vi "9149_9205_AI_64.vi"() -> (3 "Array":fxp<+/-,26,5>[](array[numeric]))   [LabVIEW 2017]
uses:
  <vilib>/rvi/eio/common/nirviEmuTemplateMethod_errors.vi
  <vilib>/eio/EIONode/EIONode.xnode
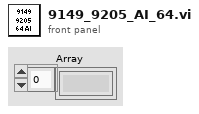
[diagram p1: front panel]
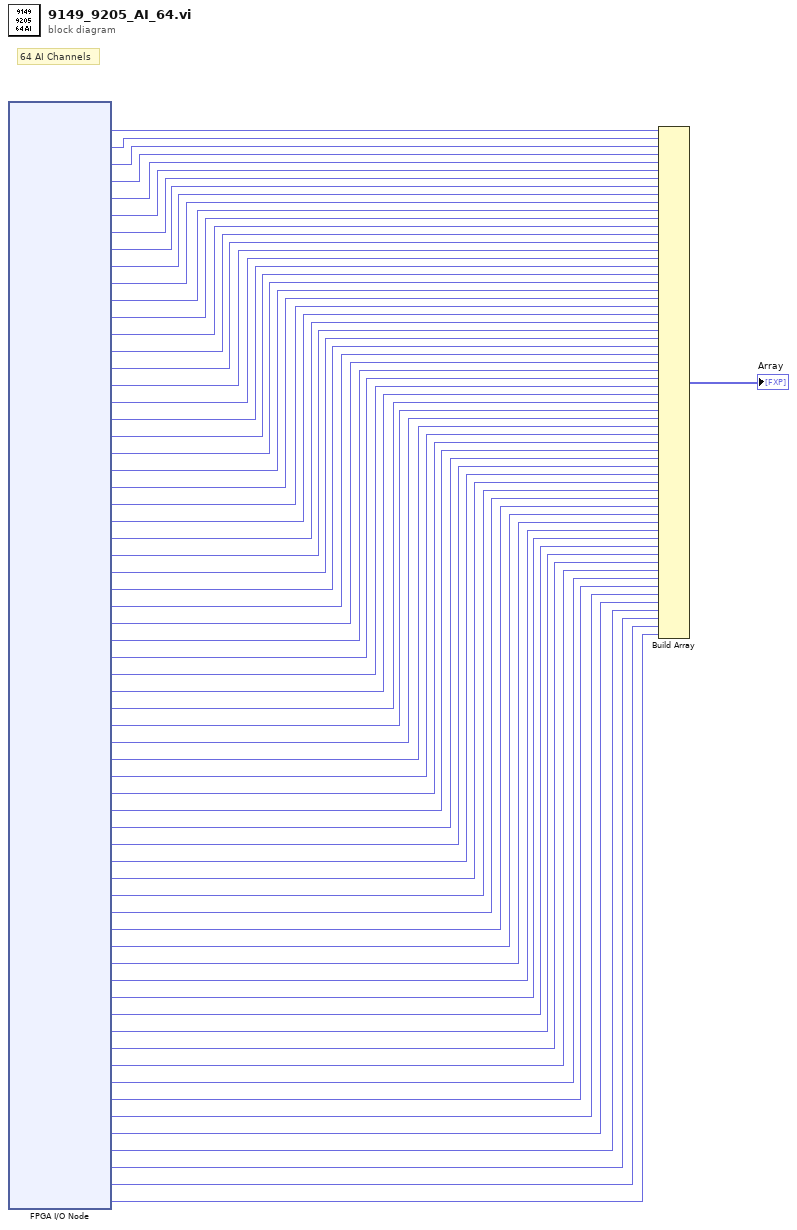
[diagram p0: block diagram]
diagram:
  # "64 AI Channels"
  n1 = xnode "FPGA I/O Node"() -> ("Mod2/AI0"=w64:fxp<+/-,26,5>, "Mod2/AI1"=w1:fxp<+/-,26,5>, "Mod2/AI2"=w2:fxp<+/-,26,5>, "Mod2/AI3"=w3:fxp<+/-,26,5>, "Mod2/AI4"=w4:fxp<+/-,26,5>, "Mod2/AI5"=w5:fxp<+/-,26,5>, "Mod2/AI6"=w6:fxp<+/-,26,5>, "Mod2/AI7"=w7:fxp<+/-,26,5>, "Mod2/AI8"=w8:fxp<+/-,26,5>, "Mod2/AI9"=w9:fxp<+/-,26,5>, "Mod2/AI10"=w10:fxp<+/-,26,5>, "Mod2/AI11"=w11:fxp<+/-,26,5>, "Mod2/AI12"=w12:fxp<+/-,26,5>, "Mod2/AI13"=w13:fxp<+/-,26,5>, "Mod2/AI14"=w14:fxp<+/-,26,5>, "Mod2/AI15"=w15:fxp<+/-,26,5>, "Mod2/AI16"=w16:fxp<+/-,26,5>, "Mod2/AI17"=w17:fxp<+/-,26,5>, "Mod2/AI18"=w18:fxp<+/-,26,5>, "Mod2/AI19"=w19:fxp<+/-,26,5>, "Mod2/AI20"=w20:fxp<+/-,26,5>, "Mod2/AI21"=w21:fxp<+/-,26,5>, "Mod2/AI22"=w22:fxp<+/-,26,5>, "Mod2/AI23"=w23:fxp<+/-,26,5>, "Mod2/AI24"=w24:fxp<+/-,26,5>, "Mod2/AI25"=w25:fxp<+/-,26,5>, "Mod2/AI26"=w26:fxp<+/-,26,5>, "Mod2/AI27"=w27:fxp<+/-,26,5>, "Mod2/AI28"=w28:fxp<+/-,26,5>, "Mod2/AI29"=w29:fxp<+/-,26,5>, "Mod2/AI30"=w30:fxp<+/-,26,5>, "Mod2/AI31"=w31:fxp<+/-,26,5>, "Mod7/AI0"=w32:fxp<+/-,26,5>, "Mod7/AI1"=w33:fxp<+/-,26,5>, "Mod7/AI2"=w34:fxp<+/-,26,5>, "Mod7/AI3"=w35:fxp<+/-,26,5>, "Mod7/AI4"=w36:fxp<+/-,26,5>, "Mod7/AI5"=w37:fxp<+/-,26,5>, "Mod7/AI6"=w38:fxp<+/-,26,5>, "Mod7/AI7"=w39:fxp<+/-,26,5>, "Mod7/AI8"=w40:fxp<+/-,26,5>, "Mod7/AI9"=w41:fxp<+/-,26,5>, "Mod7/AI10"=w42:fxp<+/-,26,5>, "Mod7/AI11"=w43:fxp<+/-,26,5>, "Mod7/AI12"=w44:fxp<+/-,26,5>, "Mod7/AI13"=w45:fxp<+/-,26,5>, "Mod7/AI14"=w46:fxp<+/-,26,5>, "Mod7/AI15"=w47:fxp<+/-,26,5>, "Mod7/AI16"=w48:fxp<+/-,26,5>, "Mod7/AI17"=w49:fxp<+/-,26,5>, "Mod7/AI18"=w50:fxp<+/-,26,5>, "Mod7/AI19"=w51:fxp<+/-,26,5>, "Mod7/AI20"=w52:fxp<+/-,26,5>, "Mod7/AI21"=w53:fxp<+/-,26,5>, "Mod7/AI22"=w54:fxp<+/-,26,5>, "Mod7/AI23"=w55:fxp<+/-,26,5>, "Mod7/AI24"=w56:fxp<+/-,26,5>, "Mod7/AI25"=w57:fxp<+/-,26,5>, "Mod7/AI26"=w58:fxp<+/-,26,5>, "Mod7/AI27"=w59:fxp<+/-,26,5>, "Mod7/AI28"=w60:fxp<+/-,26,5>, "Mod7/AI29"=w61:fxp<+/-,26,5>, "Mod7/AI30"=w62:fxp<+/-,26,5>, "Mod7/AI31"=w63:fxp<+/-,26,5>)  [unwired: 64 in, 64 out]
  n2 = Build Array(w64, w1, w2, w3, w4, w5, w6, w7, w8, w9, w10, w11, w12, w13, w14, w15, w16, w17, w18, w19, w20, w21, w22, w23, w24, w25, w26, w27, w28, w29, w30, w31, w32, w33, w34, w35, w36, w37, w38, w39, w40, w41, w42, w43, w44, w45, w46, w47, w48, w49, w50, w51, w52, w53, w54, w55, w56, w57, w58, w59, w60, w61, w62, w63) -> (→"Array":fxp<+/-,26,5>[])
